vi "Bildwechsel-Tasten beschriften.vi"(11 "Referenz":refnum<vi>) -> ()   [LabVIEW 2020, in "Bildwechsel.lvlib"]
uses:
  Bildwechsel.lvlib
  Bild-Auswahl.ctl
panel:
  in  "Bild-Auswahl":T1=enum."Grafik"
  # "Störung"
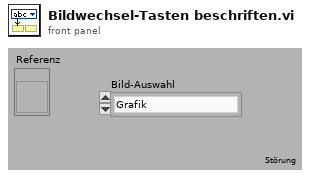
[diagram p1: front panel]
types:
  T1 = typedef "Bildwechsel.lvlib/Bild-Auswahl.ctl" = enum16{"lesen", "Initialisieren", "Beenden", "Grafik", "Anlagenübersicht", "Anlagengrenzwerte", "Log Konfig", "Gaszuordnung AO", "Erw. Konfiguration", "FT-IR  ", "Störmeldungen", "Störmeldepuffer", "Störmeldekonfig", "PNS Grenzwerte", "Statusübersicht", "Linearisierung", "ARN", "EPA Dichtheitstest", "FID", "PMA", "CalGas", "Lambda", "Interference", "Amium PNS"}
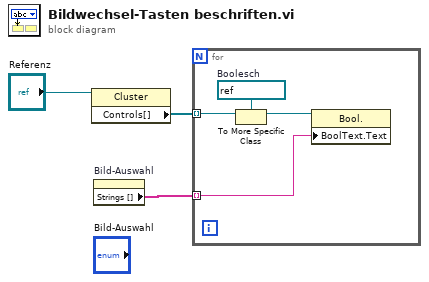
[diagram p0: block diagram]
diagram:
  n1 = property class="Cluster"(reference="Referenz") -> ("Controls[]"=w2:refnum<vi>[])  [unwired: 1 in, 2 out]
  n2 = property on="Bild-Auswahl" class="Enum (strikt)"() -> ("Strings []"=w1:string[])  [unwired: 2 in, 2 out]
  n3 = for {
    tunnel: w2 -> [w7] mode=indexing
    tunnel: w1 -> [w4] mode=indexing
    w6 = refnum<vi> refnum  # Boolesch
    n4 = To More Specific Class(target class=w6, reference=w7) -> (specific class reference=w5:refnum<vi>)  [unwired: 1 in, 1 out]
    n5 = property class="Bool."(reference=w5, "BoolText.Text"=w4) -> ()  [unwired: 1 in, 2 out]
  }
